vi "isPointScan.vi"(9 "Scan Mode":T2) -> (3 "Scan Type":T1)   [LabVIEW 2012]
uses:
  typedefs/ScanMode.ctl
  typedefs/ScanModeScanType.ctl
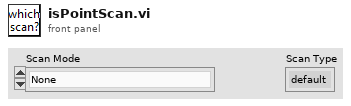
[diagram p1: front panel]
types:
  T1 = typedef "ScanModeScanType.ctl" = enum16{"default", "point scan", "grab"}
  T2 = typedef "ScanMode.ctl" = enum16{"None", "Continuous", "Point Scan (CH3 cursor)", "Point Scan Move (CH3 cursor)", "Grab", "Grab Move Stage", "Grab Move Z-stage", "Cont. Move Z-stage", "Spec Move Stage", "Spec Move Cont", "Surf Calib"}
  T3 = typedef "Move Type.ctl" = enum16{"None", "Continuous", "Discrete"}
  T4 = typedef "Scan Type.ctl" = enum16{"None", "Point", "Full Image Continuous", "Full Image Grab"}
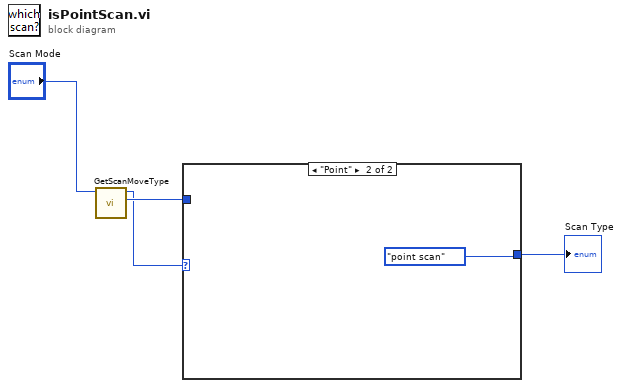
[diagram p0: block diagram]
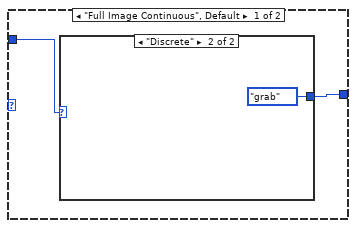
[diagram p2: hidden frame]
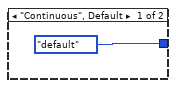
[diagram p3: hidden frame]
diagram:
  n1 = call "GetScanMoveType.vi"("Scan Mode"="Scan Mode") -> ("Move Type"=w3:T3, "Scan Type"=w2:T4)  [unwired: 8 in, 1 out]
  n2 = case shown="\"Point\"" w2 {
    tunnel: w3 -> [w6 _]
    tunnel: [w5 ScanModeScanType."point scan"] -> w1
    frame "Full Image Continuous", Default {
      n3 = case shown="\"Discrete\"" w6 {
        tunnel: [ScanModeScanType."default" ScanModeScanType."grab"] -> w5
        frame "Continuous", Default {
        }
        frame "Discrete" {
        }
      }
    }
    frame "Point" {
    }
  }
  "Scan Type" <- w1
